vi "flashV2.vi"() -> ()   [LabVIEW 2017]
panel:
  out "Numeric":i32
  out "error out 3":errorcluster={"status"=TRUE, "code"=56, "source"="UDP Read in UDP.vi->flash.vi"}
  out "index 2":i32
  out "length":i32=256
  out "字符串":string
  out "error out 2":errorcluster
  in  "error in (no error)":errorcluster
  in  "Read (TRUE)":bool
  in  "IP address":string="192.168.10.20"
  in  "display":bool=TRUE
  out "index":i32
  out "data":string
  out "String":string
  out "size (in bytes)":i64=1443180
  out "In":u8=48 format="%x"
  in  "file path (use dialog)":path=path "G:/fpga_tdc/golden/golden.runs/impl_1/top_hdl.bin"
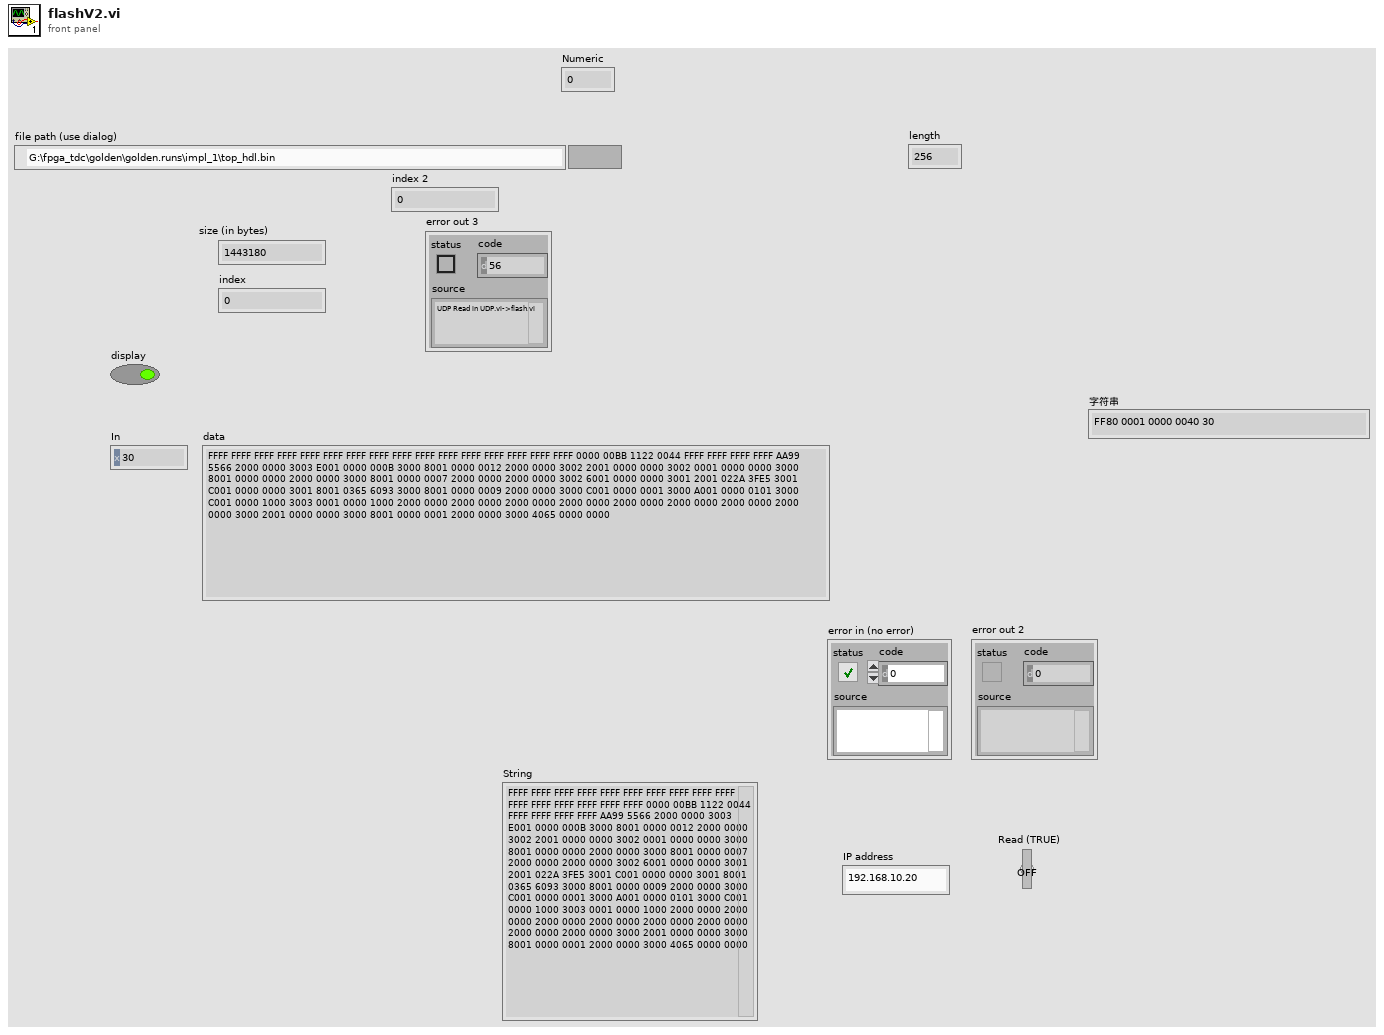
[diagram p1: front panel]
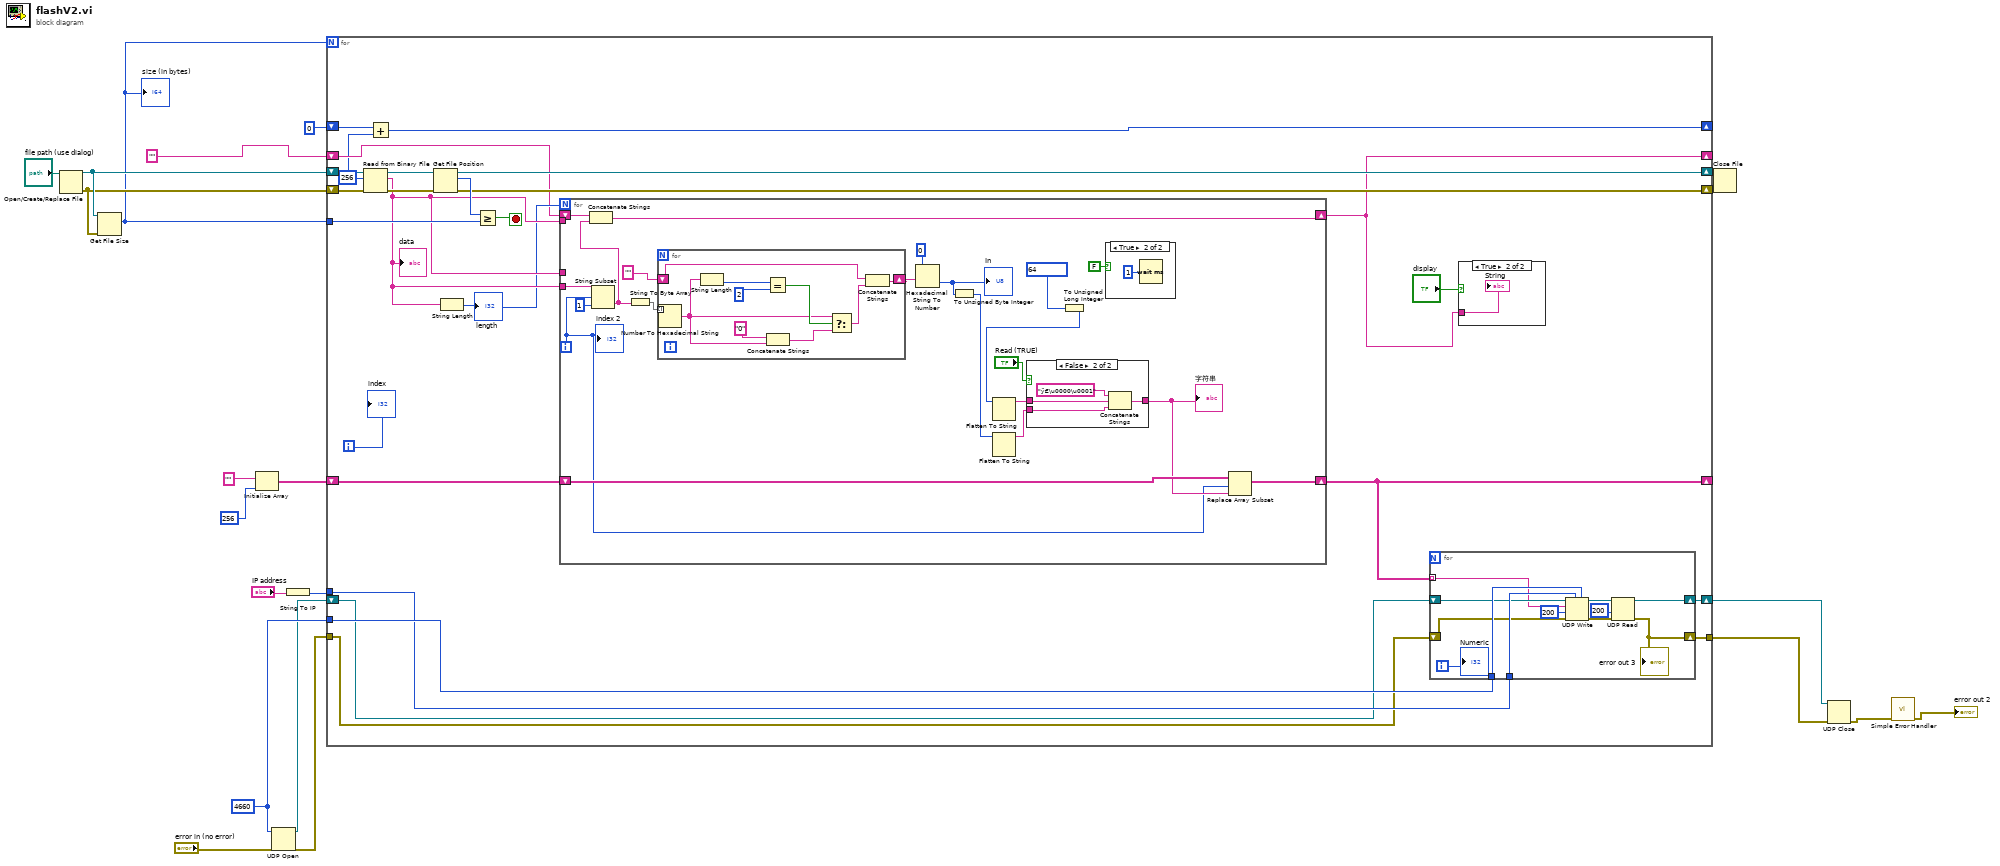
[diagram p0: block diagram]
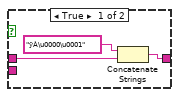
[diagram p2: hidden frame]
diagram:
  w15 = u16 4660 ("UDP port")
  n1 = Open/Create/Replace File(file path (use dialog)="file path (use dialog)") -> (refnum out=w20:refnum<file>, error out=w19:errorcluster)  [unwired: 5 in, 1 out]
  n2 = Get File Size(file=w20, error in=w19) -> (size (in bytes)=w16:i64)  [unwired: 2 out]
  "size (in bytes)" <- w16
  n3 = Initialize Array("" ("format string"), 256 ("dimension size")) -> (w3:string[])
  n4 = UDP Open(8:"error in (no error)", 11:w15) -> (port=w13:refnum<k16>, 0:w14:errorcluster)  [unwired: 3 in, 1 out]
  n5 = String To IP(1:"IP address") -> (0:w9:u32)
  n6 = for {
    N: w16 -> [_]
    tunnel: w16 -> [w42]
    shift-right: [w40] -> w18
    shift-left: w19 -> [w46]
    shift-right: [w39] -> w17
    shift-left: w20 -> [w47]
    shift-right: [w35] -> _
    shift-left: "" -> [w25]
    tunnel: w15 -> [w33]
    tunnel: w14 -> [w31]
    tunnel: [w29] -> w11
    tunnel: w9 -> [w32]
    shift-right: [w28] -> w12
    shift-left: w13 -> [w30]
    shift-right: [w26] -> _
    shift-left: w3 -> [w27]
    shift-right: [w22] -> _
    shift-left: 0 ("length (rest)") -> [w24]
    i -> [w38]
    stop <- w41 stop-if-true
    w23 = 256 ("count (1)")
    n7 = Read from Binary File(8:w46, 10:w23, 11:w47) -> (0:w44:errorcluster, 2:w36:string, 3:w45:refnum<file>)  [unwired: 3 in, 1 out]
    "data" <- w36
    n8 = Add(x=w24, y=w23) -> (x+y=w22:i32)
    n9 = Get File Position(4:w44, 7:w45) -> (0:w40:errorcluster, 2:w43:i64, 3:w39:refnum<file>)
    n10 = String Length(string=w36) -> (length=w34:i32)
    "length" <- w34
    n11 = Greater Or Equal?(x=w43, y=w42) -> (x >= y?=w41:bool)
    n12 = for {
      N: w34 -> [_]
      tunnel: w36 -> [_]
      tunnel: w36 -> [w72]
      tunnel: w36 -> [_]
      shift-right: [w69] -> w35
      shift-left: w25 -> [w70]
      shift-right: [w63] -> w26
      shift-left: w27 -> [w62]
      i -> [w60]
      n13 = String Subset(string=w72, offset (0)=w60, length (rest)=1 ("length (rest)")) -> (substring=w68:string)
      n14 = Concatenate Strings(w70, w68) -> (w69:string)
      n15 = String To Byte Array(string=w68) -> (unsigned byte array=w79:u8[])
      n16 = for {
        shift-right: [w97] -> w78
        shift-left: "" ("format string") -> [w94]
        tunnel: w79 -> [w98] mode=indexing
        n17 = Number To Hexadecimal String(2:w98) -> (0:w90:string)  [unwired: 1 in]
        n18 = String Length(string=w90) -> (length=w96:i32)
        n19 = Equal?(x=w96, y=2) -> (x = y?=w93:bool)
        n20 = Concatenate Strings("0" ("format string"), w90) -> (w92:string)
        n21 = Select(t=w90, s=w93, f=w92) -> (s? t:f=w89:string)
        n22 = Concatenate Strings(w94, w89) -> (w97:string)
      }
      n23 = Hexadecimal String To Number(string=w78, default (0uL)=u64 0 ("default (0 U32)")) -> (number=w76:u64)  [unwired: 1 in, 1 out]
      "In" <- w76
      n24 = To Unsigned Byte Integer(number=w76) -> (unsigned 8bit integer=w74:u8)
      n25 = Flatten To String(anything=w74) -> (data string=w65:string)  [unwired: 3 in, 2 out]
      n26 = To Unsigned Long Integer(number=u32 64 ("Address")) -> (unsigned 32bit integer=w73:u32)
      n27 = Flatten To String(anything=w73) -> (data string=w66:string)  [unwired: 3 in, 2 out]
      n28 = case shown="False" "Read (TRUE)" {
        tunnel: [w82 w86] -> w61
        tunnel: w66 -> [w81 w85]
        tunnel: w65 -> [_ w84]
        frame True {
          n29 = Concatenate Strings("ÿÀ\u0000\u0001" ("initial string"), w81) -> (w82:string)
        }
        frame False {
          n30 = Concatenate Strings("ÿ€\u0000\u0001" ("initial string"), w85, w84) -> (w86:string)
        }
      }
      "字符串" <- w61
      n31 = case shown="True" FALSE {
        frame False {
        }
        frame True {
          n32 = Wait (ms)(milliseconds to wait=u32 1) -> ()  [unwired: 1 out]
        }
      }
      n33 = Replace Array Subset(array=w62, new element=w61, index=w60) -> (w63:string[])
      "index 2" <- w60
    }
    n34 = for {
      tunnel: w33 -> [w56]
      tunnel: w32 -> [w55]
      shift-right: [w51] -> w29
      shift-left: w31 -> [w54]
      shift-right: [w50] -> w28
      shift-left: w30 -> [w52]
      tunnel: w26 -> [w49] mode=indexing
      i -> [w48]
      n35 = UDP Write(address=w55, port or service name=w56, connection ID=w52, data in=w49, 8:w54, 9:200 ("timeout ms (25000)")) -> (error out=w59:errorcluster, 3:w58:refnum<k16>)
      n36 = UDP Read(connection ID=w58, timeout ms (25000)=200, 8:w59) -> (error out=w51:errorcluster, 3:w50:refnum<k16>)  [unwired: 4 out]
      "error out 3" <- w51
      "Numeric" <- w48
    }
    n37 = case shown="True" "display" {
      tunnel: w35 -> [_ w99]
      frame False {
      }
      frame True {
        "String" <- w99
      }
    }
    "index" <- w38
  }
  n38 = Close File(refnum=w17, error in=w18) -> ()  [unwired: 2 out]
  n39 = UDP Close(connection ID=w12, 8:w11) -> (error out=w8:errorcluster)  [unwired: 1 out]
  n40 = call <vilib>:"Simple Error Handler.vi"("error in (no error)"=w8) -> ("error out"=→"error out 2":errorcluster)  [unwired: 4 in, 4 out]
